vi "Add Actor.vi"(8 "error in":errorcluster, 11 "Target Item":T1) -> (0 "error out":errorcluster)   [LabVIEW 2020, in "Add Actor.lvlib"]
uses:
  Add Actor.lvlib
  <resource>/Framework/Providers/API/mxLvNIIM.ctl
  Classes/INI Store/INI Store.lvclass
  C:/justACS/Actor Framework/Providers/AddActor/Classes/Actor Store/Actor Store.lvclass
  Classes/Target Store/Target Store.lvclass
  Localized Strings.vi
  MessageMakerProvider/AFPP Shared/AFPP Shared.lvlib
  C:/justACS/Actor Framework/Providers/AddActor/Classes/INI Store/INI Store.lvclass
  C:/justACS/Actor Framework/Providers/AddActor/Classes/Target Store/Target Store.lvclass
panel:
  out "Path Display":string
  in  "Path":path caption="Save files to..."
  in  "Remove Actor":bool
  in  "Inherit from:":string(combo)
  in  "Cancel Button":bool
  in  "OK Button":bool
  in  "Name of Actor":string
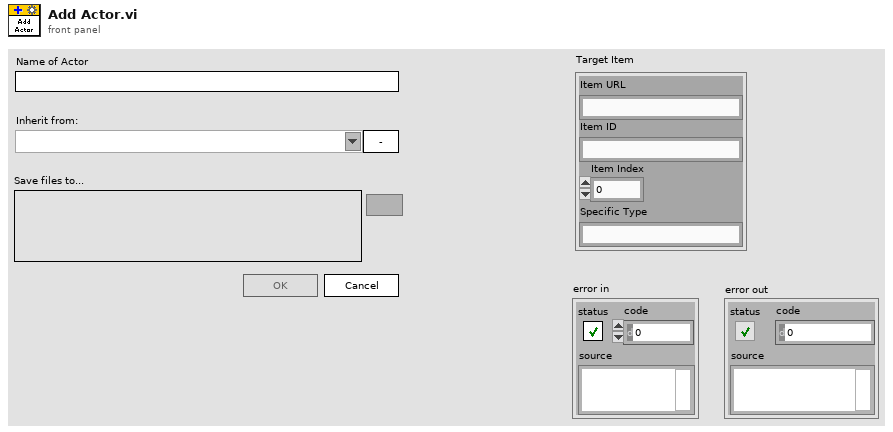
[diagram p1: front panel]
types:
  T1 = typedef "mxLvNIIM.ctl" = cluster{"Item URL":string, "Item ID":string, "Item Index":i32, "Specific Type":string}
  T2 = enum8{"Enabled", "Disabled", "Disabled and Grayed Out"}
  T3 = enum32{"Invalid", "Standard", "Closed", "Hidden", "Minimized", "Maximized"}
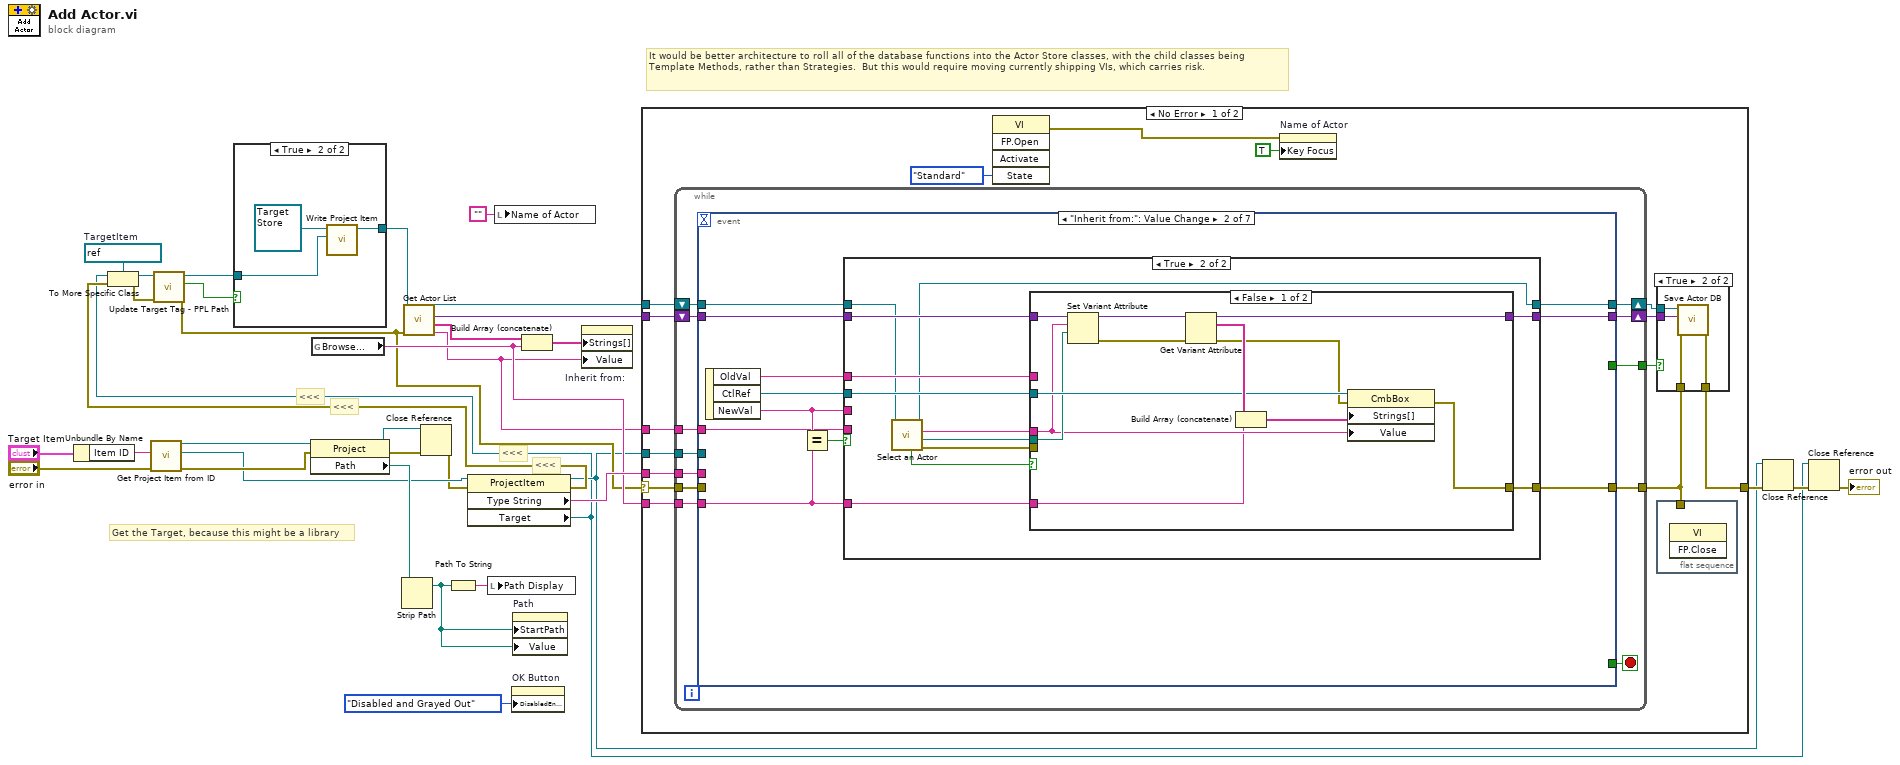
[diagram p0: block diagram]
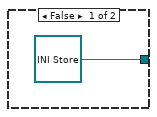
[diagram p2: hidden frame]
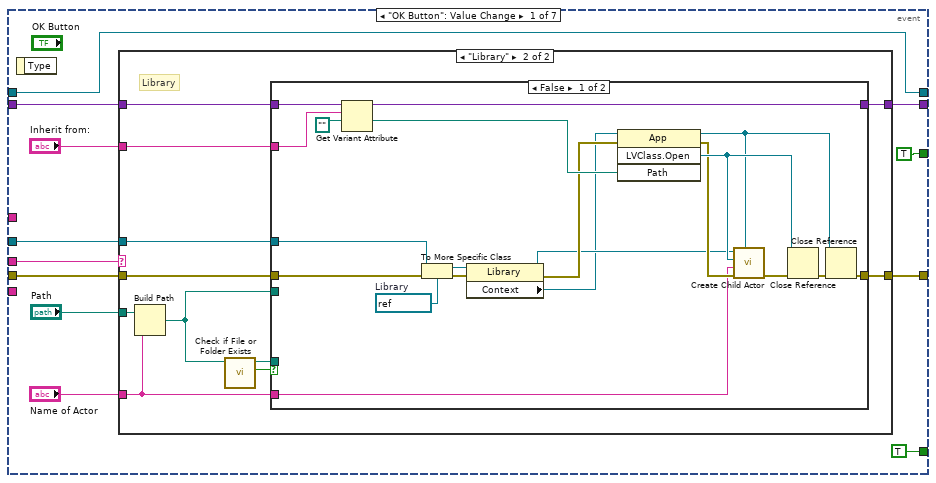
[diagram p3: hidden frame]
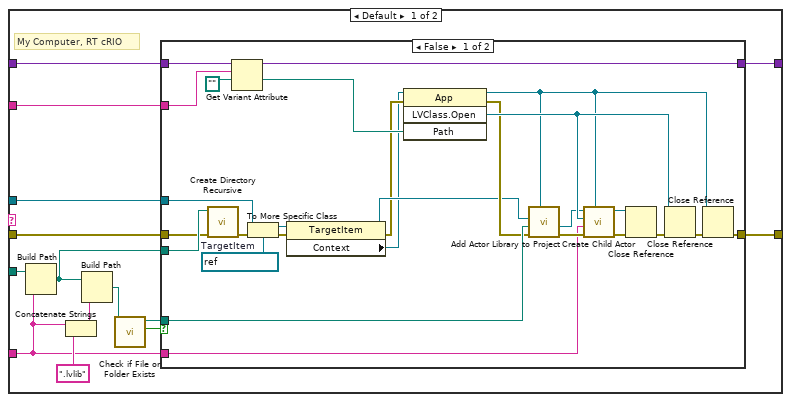
[diagram p4: hidden frame]
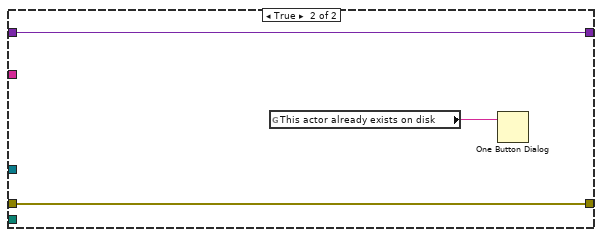
[diagram p5: hidden frame]
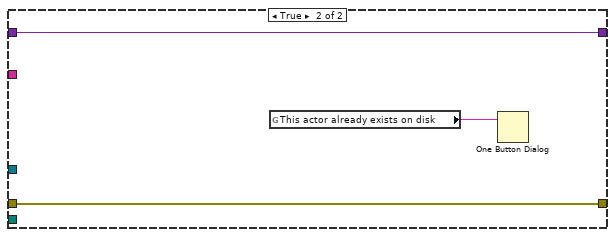
[diagram p6: hidden frame]
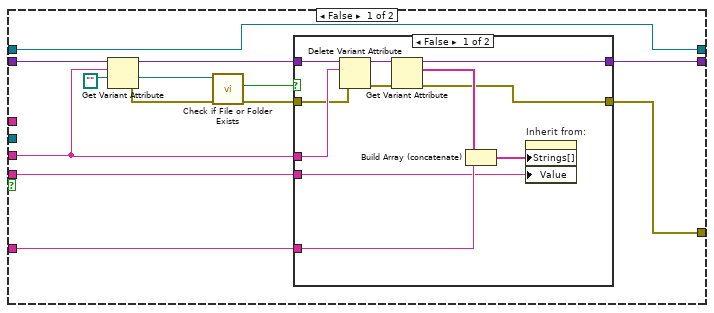
[diagram p7: hidden frame]
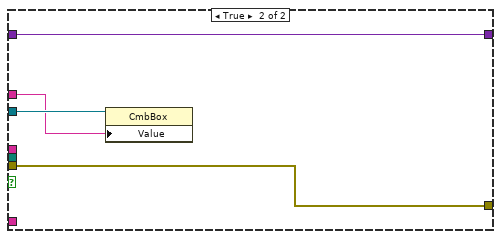
[diagram p9: hidden frame]
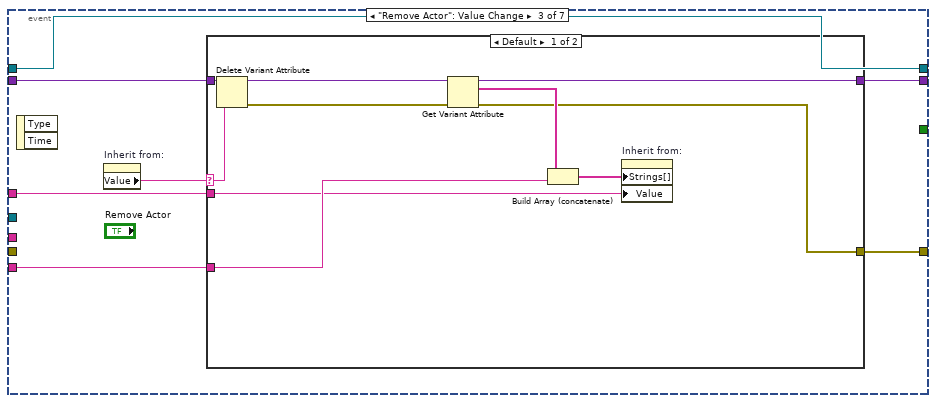
[diagram p10: hidden frame]
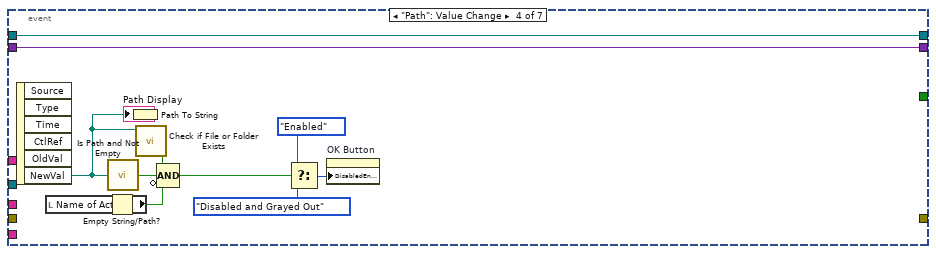
[diagram p12: hidden frame]
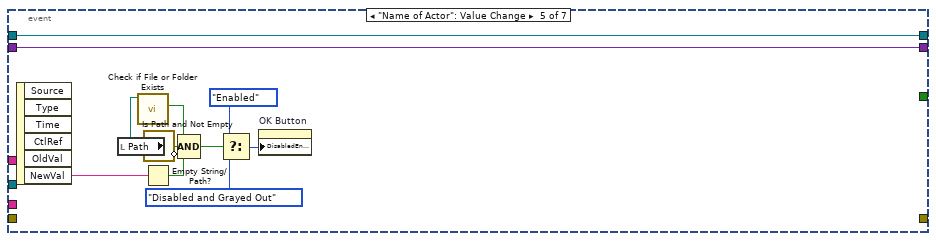
[diagram p13: hidden frame]
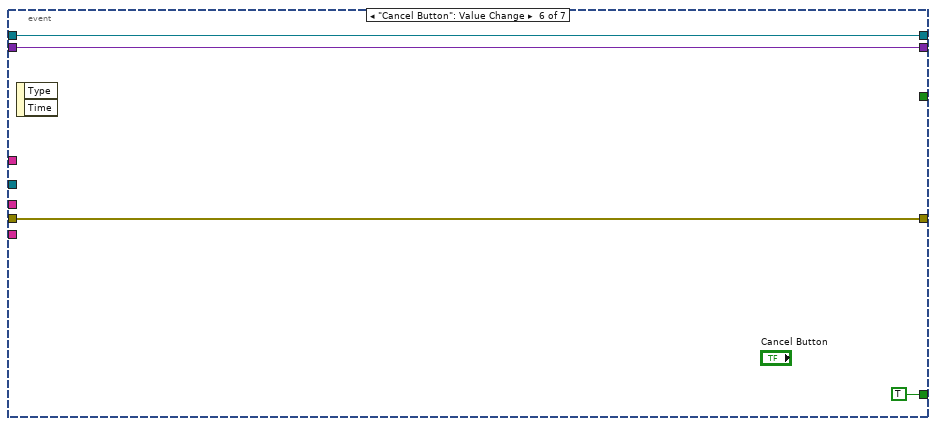
[diagram p14: hidden frame]
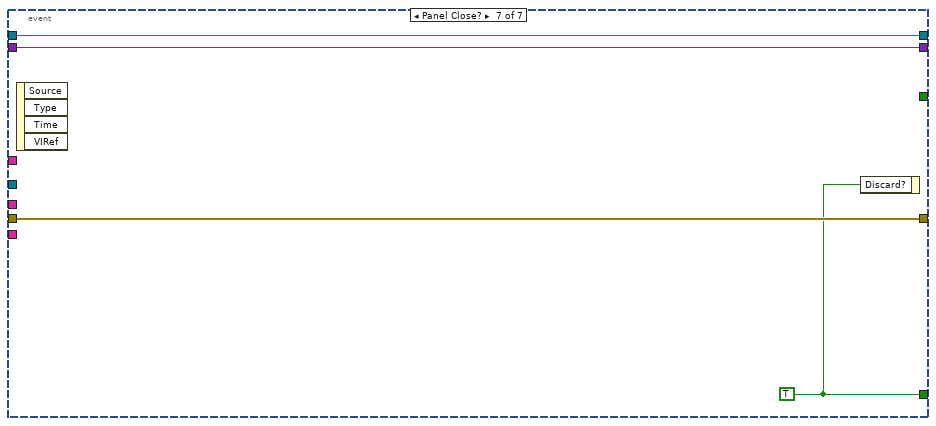
[diagram p15: hidden frame]
diagram:
  w8 = refnum<vi> refnum  # TargetItem
  # "Get the Target, because this might be a library"
  # "<<<"
  # "<<<"
  # "<<<"
  # "<<<"
  # "It would be better architecture to roll all of the database functions into the Actor Store classes, with the child classes being Template Methods, rather than Strategies.  But this would require moving currently shipping VIs, which carries risk."
  n1 = Unbundle By Name("Target Item") -> ("Item ID"=w1:string)
  n2 = call "Get Project Item from ID.vi"("error in (no error)"="error in", "Item ID"=w1) -> ("error out"=w28:errorcluster, "Project Item"=w23:refnum<vi>, "Project out"=w27:refnum<vi>)  [unwired: 7 in]
  n3 = property class="Project"(reference=w27, error in=w28) -> (reference out=w17:refnum<vi>, error out=w19:errorcluster, "Path"=w30:path)
  n4 = global read "Localized Strings.vi" "Browse..."() -> (w24:string)
  n5 = Strip Path(path=w30) -> (stripped path=w21:path)  [unwired: 1 out]
  n6 = Close Reference(reference=w17, error in (no error)=w19) -> (error out=w18:errorcluster)
  n7 = Path To String(path=w21) -> (string=w22:string)
  n8 = property class="ProjectItem"(reference=w23, error in=w18) -> (reference out=w3:refnum<vi>, error out=w5:errorcluster, "Type String"=w29:string, "Target"=w2:refnum<vi>)
  n9 = To More Specific Class(target class=w8, reference=w2, error in=w5) -> (specific class reference=w7:refnum<vi>, error out=w6:errorcluster)
  n10 = call "Update Target Tag - PPL Path.vi"("error in (no error)"=w6, "Target"=w7) -> ("error out"=w9:errorcluster, "Found PPL?"=w16:bool, "dup Target"=w14:refnum<vi>)  [unwired: 7 in]
  n11 = case shown="True" w16 {
    tunnel: [refnum<class "INI Store.lvclass"> refnum ("Add Actor.lvlib:INI Store.lvclass") w38] -> w15
    tunnel: w14 -> [_ w36]
    frame False {
    }
    frame True {
      n12 = call-dynamic "Write Project Item.vi"("Project Item"=w36, "Target Store in"=refnum<class "Target Store.lvclass"> refnum) -> ("Target Store out"=w38:refnum<class "Target Store.lvclass">)  [unwired: 9 in]
    }
  }
  n13 = call "Get Actor List.vi"("error in (no error)"=w9, "Actor Store"=w15) -> ("Actor Label"=w20:string, "Actors"=w12:string[], "Actor Paths"=w34:variant, "Actor Store"=w13:refnum<class "Actor Store.lvclass">)  [unwired: 6 in]
  n14 = local write "Path Display"(w22) -> ()
  n15 = local write "Name of Actor"("" ("Name of Actor")) -> ()
  n16 = property on="OK Button" class="Bool"("DisabledEnum"=T2."Disabled and Grayed Out" ("Disabled")) -> ()  [unwired: 2 in, 2 out]
  n17 = property on="Path" class="Path"("StartPath"=w21, "Value"=w21) -> ()  [unwired: 2 in, 2 out]
  n18 = Build Array (concatenate)(w12, w24) -> (w33:string[])
  n19 = property on="Inherit from:" class="CmbBox"("Strings[]"=w33, "Value"=w20) -> ()  [unwired: 2 in, 2 out]
  n20 = case shown="No Error" w9 {
    selector: w9 -> [w53 w275]
    tunnel: [w47 w275] -> w10
    tunnel: w34 -> [w52 _]
    tunnel: w29 -> [w51 _]
    tunnel: w3 -> [w50 _]
    tunnel: w24 -> [w49 _]
    tunnel: w20 -> [w45 _]
    tunnel: w13 -> [w44 _]
    frame No Error {
      n21 = while {
        tunnel: [w65] -> w41
        tunnel: w53 -> [w64]
        shift-right: [w61] -> w48
        shift-left: w52 -> [w62]
        tunnel: w51 -> [w60]
        tunnel: w50 -> [w59]
        tunnel: w49 -> [w58]
        tunnel: [w57] -> w46
        tunnel: w45 -> [w56]
        shift-right: [w54] -> w43
        shift-left: w44 -> [w55]
        stop <- w63 stop-if-true
        n22 = event shown="[1] \"Inherit from:\": Value Change" {
          selector: _ -> [_ _ _ _ _ _ _]
          dyn-events: _ -> [_ _ _ _ _ _ _]
          timeout: _ -> [_ _ _ _ _ _ _]
          tunnel: w64 -> [w71 _ _ _ _ w264 w269]
          tunnel: [w72 w166 w224 _ _ w264 w269] -> w65
          tunnel: [TRUE _ _ _ _ TRUE w267] -> w63
          tunnel: w62 -> [w75 w165 w226 w247 w254 w263 w268]
          tunnel: [w73 w164 w225 w247 w254 w263 w268] -> w61
          tunnel: w60 -> [w70 _ _ _ _ _ _]
          tunnel: w59 -> [w69 _ _ _ _ _ _]
          tunnel: w58 -> [_ w160 w223 _ _ _ _]
          tunnel: [TRUE _ _ _ _ _ _] -> w57
          tunnel: w56 -> [_ w159 w222 _ _ _ _]
          tunnel: w55 -> [w66 w157 w221 w239 w251 w262 w266]
          tunnel: [w66 w156 w221 w239 w251 w262 w266] -> w54
          event "OK Button": Value Change {
            n23 = event-data() -> ()  [unwired: 1 in, 1 out]
            n24 = case shown="\"Library\"" w70 {
              tunnel: "Path" -> [w91 w132]
              tunnel: "Name of Actor" -> [w79 w123]
              tunnel: w75 -> [w90 w131]
              tunnel: "Inherit from:" -> [w89 w130]
              tunnel: [w88 w129] -> w73
              tunnel: [w85 w127] -> w72
              tunnel: w71 -> [w84 w126]
              tunnel: w69 -> [w82 w124]
              frame Default {
                # "My Computer, RT cRIO"
                n25 = Build Path(base path=w91, name or relative path=w79) -> (appended path=w87:path)
                n26 = Concatenate Strings(w79, ".lvlib" ("string")) -> (w80:string)
                n27 = Build Path(base path=w87, name or relative path=w80) -> (appended path=w78:path)
                n28 = call <vilib>:"Check if File or Folder Exists.vi"("path"=w78) -> ("file or folder exists?"=w83:bool, "dup path"=w86:path)  [unwired: 8 in, 1 out]
                n29 = case shown="False" w83 {
                  tunnel: w79 -> [w102 _]
                  tunnel: w90 -> [w117 w121]
                  tunnel: w89 -> [w116 _]
                  tunnel: [w115 w121] -> w88
                  tunnel: w87 -> [w101 _]
                  tunnel: w86 -> [w112 _]
                  tunnel: [w103 w120] -> w85
                  tunnel: w84 -> [w100 w120]
                  tunnel: w82 -> [w106 _]
                  frame False {
                    w111 = refnum<vi> refnum  # TargetItem
                    n30 = call <vilib>:"Create Directory Recursive.vi"("error in (no error)"=w100, "directory"=w101) -> ("error out"=w99:errorcluster)  [unwired: 3 in, 2 out]
                    n31 = Get Variant Attribute(Variant=w117, name=w116, default value (empty Variant)=path "") -> (duplicate Variant=w115:variant, value=w114:path)  [unwired: 1 in, 2 out]
                    n32 = To More Specific Class(target class=w111, reference=w106, error in=w99) -> (specific class reference=w98:refnum<vi>, error out=w96:errorcluster)
                    n33 = property class="TargetItem"(reference=w98, error in=w96) -> (reference out=w97:refnum<vi>, error out=w95:errorcluster, "Context"=w94:refnum<vi>)
                    n34 = invoke class="App" method="LVClass.Open"(reference=w94, error in=w95, "Path"=w114) -> (reference out=w93:refnum<vi>, error out=w105:errorcluster, "LVClass.Open"=w118:refnum<vi>)  [unwired: 1 in, 1 out]
                    n35 = call "Add Actor Library to Project.vi"("Application"=w93, "error in (no error)"=w105, "Library Path"=w112, "Target Item"=w97) -> ("error out"=w110:errorcluster, "Library out"=w109:refnum<vi>)  [unwired: 6 in]
                    n36 = call "Create Child Actor.vi"("App Inst"=w93, "error in (no error)"=w110, "Actor Name"=w102, "Parent Class"=w118, "Library in"=w109) -> ("error out"=w108:errorcluster, "Library out"=w107:refnum<vi>)  [unwired: 5 in]
                    n37 = Close Reference(reference=w107, error in (no error)=w108) -> (error out=w92:errorcluster)
                    n38 = Close Reference(reference=w118, error in (no error)=w92) -> (error out=w104:errorcluster)
                    n39 = Close Reference(reference=w93, error in (no error)=w104) -> (error out=w103:errorcluster)
                  }
                  frame True {
                    n40 = global read "Localized Strings.vi" "This actor already exists on disk"() -> (w119:string)
                    n41 = One Button Dialog(message=w119) -> ()  [unwired: 1 in, 1 out]
                  }
                }
              }
              frame "Library" {
                # "Library"
                n42 = Build Path(base path=w132, name or relative path=w123) -> (appended path=w122:path)
                n43 = call <vilib>:"Check if File or Folder Exists.vi"("path"=w122) -> ("file or folder exists?"=w125:bool, "dup path"=w128:path)  [unwired: 8 in, 1 out]
                n44 = case shown="False" w125 {
                  tunnel: w123 -> [w141 _]
                  tunnel: w131 -> [w151 w155]
                  tunnel: w130 -> [w150 _]
                  tunnel: [w149 w155] -> w129
                  tunnel: w122 -> [_ _]
                  tunnel: w128 -> [_ _]
                  tunnel: [w142 w154] -> w127
                  tunnel: w126 -> [w140 w154]
                  tunnel: w124 -> [w145 _]
                  frame False {
                    w146 = refnum<vi> refnum  # Library
                    n45 = Get Variant Attribute(Variant=w151, name=w150, default value (empty Variant)=path "") -> (duplicate Variant=w149:variant, value=w148:path)  [unwired: 1 in, 2 out]
                    n46 = To More Specific Class(target class=w146, reference=w145, error in=w140) -> (specific class reference=w138:refnum<vi>, error out=w136:errorcluster)
                    n47 = property class="Library"(reference=w138, error in=w136) -> (reference out=w137:refnum<vi>, error out=w139:errorcluster, "Context"=w135:refnum<vi>)
                    n48 = invoke class="App" method="LVClass.Open"(reference=w135, error in=w139, "Path"=w148) -> (reference out=w134:refnum<vi>, error out=w144:errorcluster, "LVClass.Open"=w152:refnum<vi>)  [unwired: 1 in, 1 out]
                    n49 = call "Create Child Actor.vi"("App Inst"=w134, "error in (no error)"=w144, "Actor Name"=w141, "Parent Class"=w152, "Library in"=w137) -> ("error out"=w133:errorcluster)  [unwired: 5 in, 1 out]
                    n50 = Close Reference(reference=w152, error in (no error)=w133) -> (error out=w143:errorcluster)
                    n51 = Close Reference(reference=w134, error in (no error)=w143) -> (error out=w142:errorcluster)
                  }
                  frame True {
                    n52 = global read "Localized Strings.vi" "This actor already exists on disk"() -> (w153:string)
                    n53 = One Button Dialog(message=w153) -> ()  [unwired: 1 in, 1 out]
                  }
                }
              }
            }
          }
          event "Inherit from:": Value Change {
            n54 = event-data() -> ("OldVal"=w158:string, "CtlRef"=w163:refnum<vi>, "NewVal"=w161:string)  [unwired: 1 in]
            n55 = Equal?(x=w161, y=w160) -> (x = y?=w162:bool)
            n56 = case shown="True" w162 {
              tunnel: [w172 w198] -> w166
              tunnel: w165 -> [w179 w200]
              tunnel: [w173 w199] -> w164
              tunnel: w163 -> [_ w197]
              tunnel: w161 -> [w170 _]
              tunnel: w160 -> [w169 w196]
              tunnel: w159 -> [w168 _]
              tunnel: w158 -> [_ w195]
              tunnel: w157 -> [w167 w194]
              tunnel: [w167 w193] -> w156
              frame False {
                n57 = Get Variant Attribute(Variant=w179, name=w170, default value (empty Variant)=path "") -> (duplicate Variant=w176:variant, value=w178:path, error out=w175:errorcluster)  [unwired: 1 in, 1 out]
                n58 = call <vilib>:"Check if File or Folder Exists.vi"("error in (no error)"=w175, "path"=w178) -> ("error out"=w174:errorcluster, "file or folder exists?"=w171:bool)  [unwired: 7 in, 1 out]
                n59 = case shown="False" w171 {
                  tunnel: w176 -> [w190 w192]
                  tunnel: w170 -> [w189 _]
                  tunnel: w174 -> [w188 w191]
                  tunnel: [w183 w192] -> w173
                  tunnel: [w182 w191] -> w172
                  tunnel: w169 -> [w181 _]
                  tunnel: w168 -> [w180 _]
                  frame False {
                    n60 = Delete Variant Attribute(4:w188, 6:w189, 7:w190) -> (0:w184:errorcluster, 3:w187:variant)  [unwired: 1 out]
                    n61 = Get Variant Attribute(Variant=w187, error in=w184) -> (duplicate Variant=w183:variant, names=w185:string[], error out=w182:errorcluster)  [unwired: 2 in, 1 out]
                    n62 = Build Array (concatenate)(w185, w181) -> (w186:string[])
                    n63 = property on="Inherit from:" class="CmbBox"("Strings[]"=w186, "Value"=w180) -> ()  [unwired: 2 in, 2 out]
                  }
                  frame True {
                  }
                }
              }
              frame True {
                n64 = call "Select an Actor.vi"("Actor Store"=w194) -> ("error out"=w204:errorcluster, "Path to Actor"=w203:path, "Name of Actor"=w202:string, "Actor Store"=w193:refnum<class "Actor Store.lvclass">, "Cancelled"=w201:bool)  [unwired: 6 in]
                n65 = case shown="False" w201 {
                  tunnel: w202 -> [w206 _]
                  tunnel: w203 -> [w208 _]
                  tunnel: w204 -> [_ w219]
                  tunnel: w200 -> [w210 w220]
                  tunnel: [w213 w220] -> w199
                  tunnel: [w211 w219] -> w198
                  tunnel: w197 -> [w215 w218]
                  tunnel: w196 -> [w205 _]
                  tunnel: w195 -> [_ w217]
                  frame False {
                    n66 = Set Variant Attribute(Variant=w210, name=w206, value=w208) -> (Variant out=w209:variant, error out=w207:errorcluster)  [unwired: 1 in, 1 out]
                    n67 = Get Variant Attribute(Variant=w209, error in=w207) -> (duplicate Variant=w213:variant, names=w216:string[], error out=w212:errorcluster)  [unwired: 2 in, 1 out]
                    n68 = Build Array (concatenate)(w216, w205) -> (w214:string[])
                    n69 = property class="CmbBox"(reference=w215, error in=w212, "Strings[]"=w214, "Value"=w206) -> (error out=w211:errorcluster)  [unwired: 1 out]
                  }
                  frame True {
                    n70 = property class="CmbBox"(reference=w218, "Value"=w217) -> ()  [unwired: 1 in, 2 out]
                  }
                }
              }
            }
          }
          event "Remove Actor": Value Change {
            n71 = event-data() -> ()  [unwired: 1 in, 2 out]
            n72 = property on="Inherit from:" class="CmbBox"() -> ("Value"=w227:string)  [unwired: 2 in, 2 out]
            n73 = case shown="Default" w227 {
              selector: w227 -> [w233 _]
              tunnel: w226 -> [w236 w238]
              tunnel: [w235 w238] -> w225
              tunnel: [w234 _] -> w224
              tunnel: w223 -> [w229 _]
              tunnel: w222 -> [w228 _]
              frame Default {
                n74 = Delete Variant Attribute(6:w233, 7:w236) -> (0:w230:errorcluster, 3:w231:variant)  [unwired: 1 in, 1 out]
                n75 = Get Variant Attribute(Variant=w231, error in=w230) -> (duplicate Variant=w235:variant, names=w237:string[], error out=w234:errorcluster)  [unwired: 2 in, 1 out]
                n76 = Build Array (concatenate)(w237, w229) -> (w232:string[])
                n77 = property on="Inherit from:" class="CmbBox"("Strings[]"=w232, "Value"=w228) -> ()  [unwired: 2 in, 2 out]
              }
              frame "Actor", "Browse..." {
              }
            }
          }
          event "Path": Value Change {
            n78 = event-data() -> ("NewVal"=w240:path)  [unwired: 1 in, 5 out]
            n79 = local read "Name of Actor"() -> (w246:string)
            n80 = Empty String/Path?(string/path=w246) -> (empty?=w245:bool)
            n81 = call <vilib>:"Is Path and Not Empty.vi"("path"=w240) -> ("Is Path and Not Empty?"=w244:bool)  [unwired: 4 in]
            n82 = Path To String(path=w240) -> (string=→"Path Display":string)
            n83 = call <vilib>:"Check if File or Folder Exists.vi"("path"=w240) -> ("file or folder exists?"=w241:bool)  [unwired: 8 in, 2 out]
            n84 = Compound Arithmetic op=AND(w241, w244, invert w245) -> (w243:bool)
            n85 = Select(t=T2."Enabled" ("Disabled"), s=w243, f=T2."Disabled and Grayed Out" ("Disabled")) -> (s? t:f=w249:T2)
            n86 = property on="OK Button" class="Bool"("DisabledEnum"=w249) -> ()  [unwired: 2 in, 2 out]
          }
          event "Name of Actor": Value Change {
            n87 = event-data() -> ("NewVal"=w255:string)  [unwired: 1 in, 5 out]
            n88 = local read "Path"() -> (w252:path)
            n89 = call <vilib>:"Check if File or Folder Exists.vi"("path"=w252) -> ("file or folder exists?"=w253:bool)  [unwired: 8 in, 2 out]
            n90 = Empty String/Path?(string/path=w255) -> (empty?=w258:bool)
            n91 = call <vilib>:"Is Path and Not Empty.vi"("path"=w252) -> ("Is Path and Not Empty?"=w257:bool)  [unwired: 4 in]
            n92 = Compound Arithmetic op=AND(w253, w257, invert w258) -> (w256:bool)
            n93 = Select(t=T2."Enabled" ("Disabled"), s=w256, f=T2."Disabled and Grayed Out" ("Disabled")) -> (s? t:f=w260:T2)
            n94 = property on="OK Button" class="Bool"("DisabledEnum"=w260) -> ()  [unwired: 2 in, 2 out]
          }
          event "Cancel Button": Value Change {
            n95 = event-data() -> ()  [unwired: 1 in, 2 out]
          }
          event Panel Close? {
            w267 = TRUE
            n96 = event-data() -> ()  [unwired: 1 in, 4 out]
            n97 = event-data("Discard?"=w267) -> ()  [unwired: 1 in, 1 out]
          }
        }
      }
      n98 = invoke class="VI" method="FP.Open"("State"=T3."Standard") -> (error out=w39:errorcluster)  [unwired: 4 in, 4 out]
      n99 = property on="Name of Actor" class="Str"(error in=w39, "Key Focus"=TRUE) -> ()  [unwired: 1 in, 2 out]
      n100 = case shown="True" w46 {
        tunnel: w48 -> [_ w272]
        tunnel: [w270 w274] -> w47
        tunnel: w41 -> [w270 w273]
        tunnel: w43 -> [_ w271]
        frame False {
        }
        frame True {
          n101 = call "Save Actor DB.vi"("error in (no error)"=w273, "Actor DB"=w272, "Actor Store"=w271) -> ("error out"=w274:errorcluster)  [unwired: 6 in, 2 out]
        }
      }
      n102 = flat-sequence {
        tunnel: w41 -> [_]
        frame #0 {
          n103 = invoke class="VI" method="FP.Close"() -> ()  [unwired: 3 in, 3 out]
        }
      }
    }
    frame Error {
    }
  }
  n104 = Close Reference(reference=w3, error in (no error)=w10) -> (error out=w11:errorcluster)
  n105 = Close Reference(reference=w2, error in (no error)=w11) -> (error out=→"error out":errorcluster)
